vi "LogFile Schreiben.vi"(6 "Aktion":T1, 10 "LogFile erstellen?":bool) -> (0 "error out":errorcluster, 1 "Pfad+Name":path, 2 "Sequence":u32, 3 "LogFile schreiben ?":bool)   [LabVIEW 2020, in "LogKonfig.lvlib"]
uses:
  LogKonfig.lvlib
  Aktionen LogFile schreiben.ctl
  Aktionen Logdatei erstellen.ctl
  Log Sequence FGV Aktion.ctl
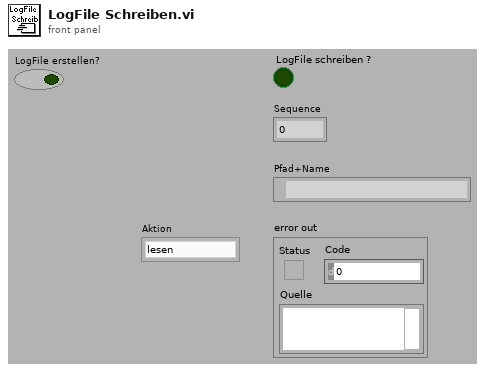
[diagram p1: front panel]
types:
  T1 = typedef "LogKonfig.lvlib/Aktionen LogFile schreiben.ctl" = enum16{"lesen", "schreiben", "initialisieren"}
  T2 = typedef "LogKonfig.lvlib/Log Sequence FGV Aktion.ctl" = enum16{"initialisieren", "lesen", "schreiben", "laden", "speichern", "übertragen"}
  T3 = typedef "LogKonfig.lvlib/Aktionen Logdatei erstellen.ctl" = enum16{"lesen", "Logdatei erstellen NEU", "Name NEU", "Pfad NEU", "Log Stop", "max Size"}
  T4 = typedef "TOOLweb Interface.lvlib/Typdefinitionen.lvlib/TOOLweb Signalverläufe.ctl" = waveform(dbl)[]
  T5 = cluster{"Index Array":i32[], "Namen Array":string[], "Spektrum File Name":bool}
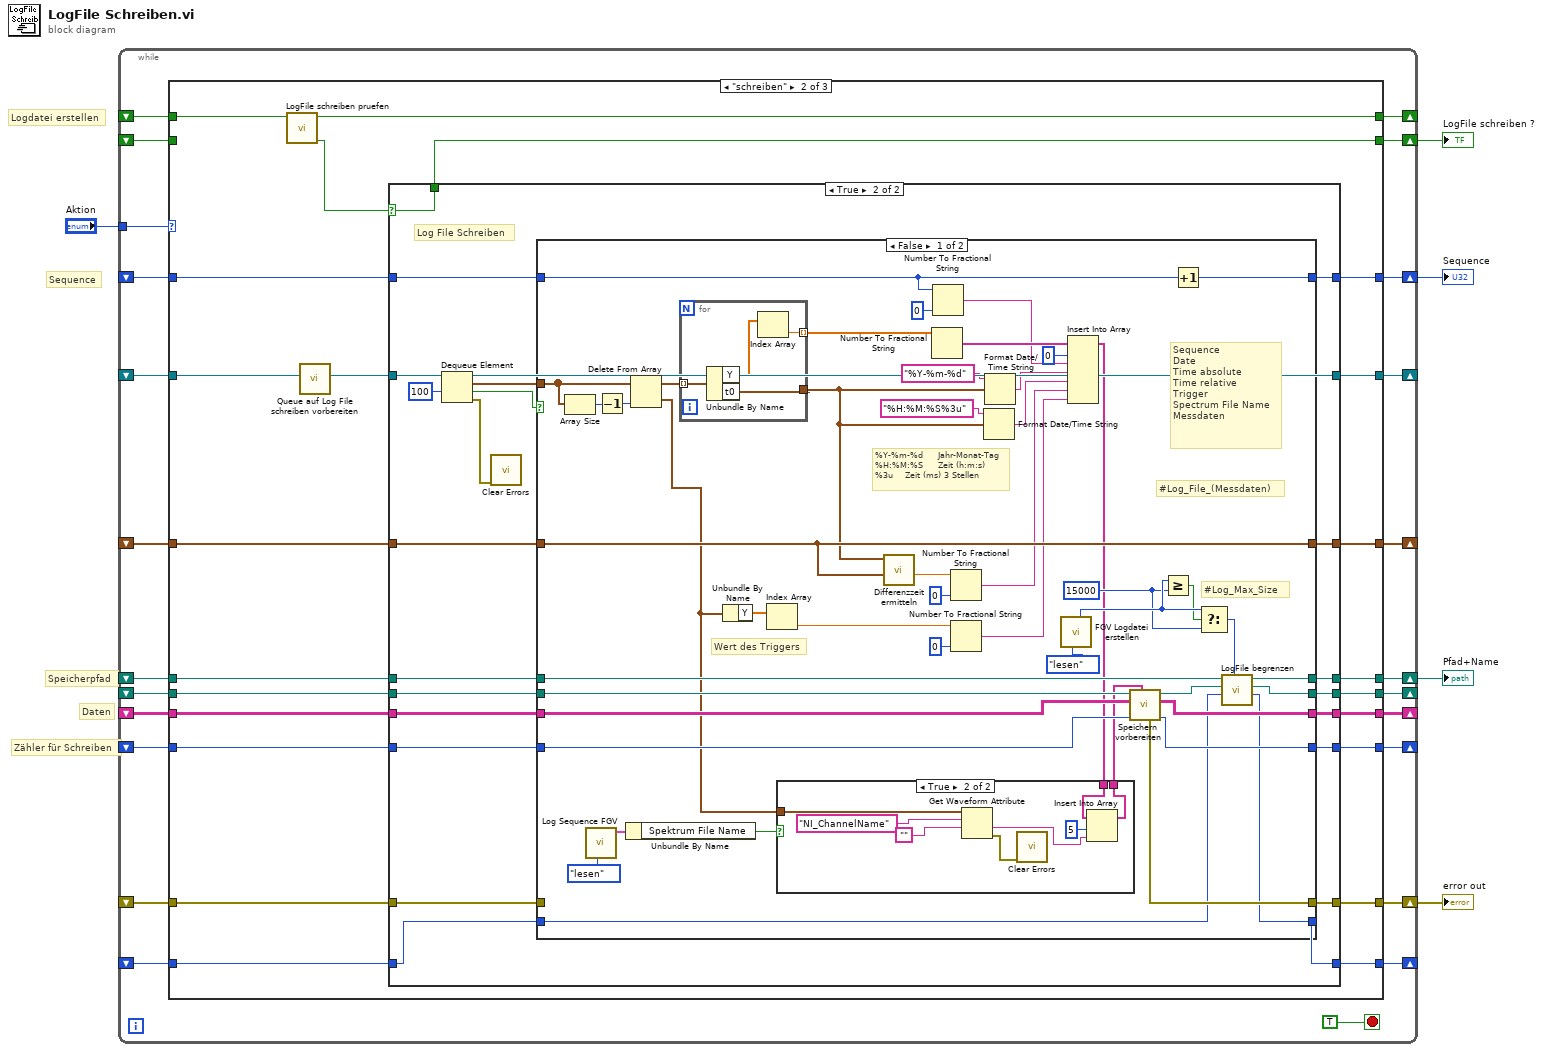
[diagram p0: block diagram]
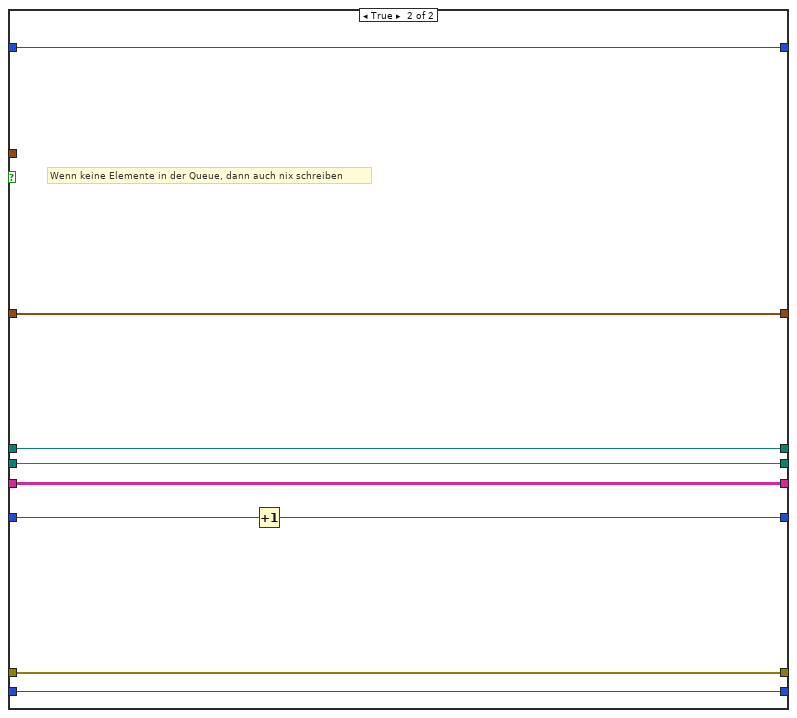
[diagram p5: hidden frame]
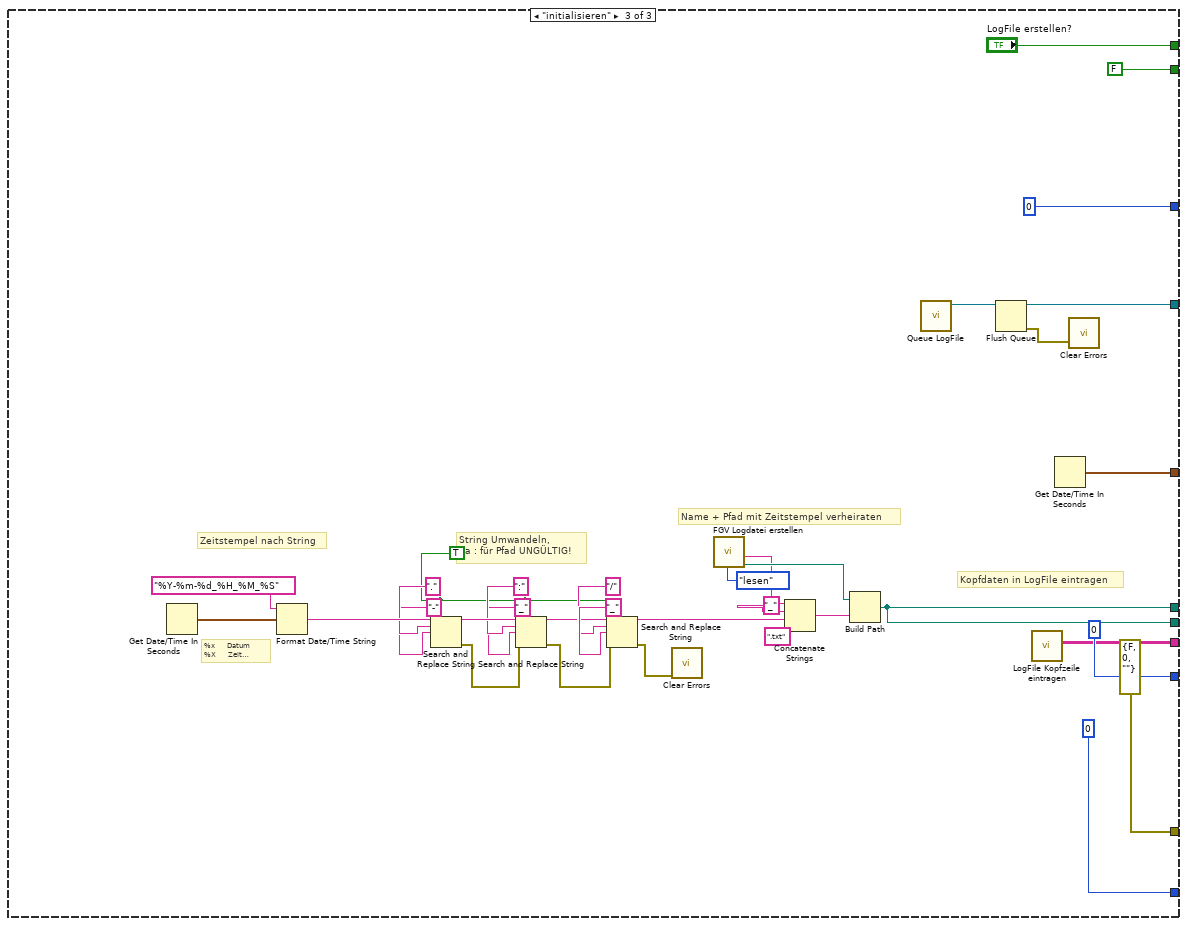
[diagram p6: hidden frame]
diagram:
  # "Zähler für Schreiben"
  # "Daten"
  # "Speicherpfad"
  # "Logdatei erstellen"
  # "Sequence"
  n1 = while {
    shift-right: [w28] -> _
    shift-left: _ -> [w29]
    shift-right: [w27] -> _
    shift-left: _ -> [w26]
    shift-right: [w25] -> _
    shift-left: _ -> [w24]
    shift-right: [w22] -> w3
    shift-left: _ -> [w23]
    tunnel: "Aktion" -> [w14]
    shift-right: [w20] -> _
    shift-left: _ -> [w19]
    shift-right: [w18] -> w4
    shift-left: _ -> [w17]
    shift-right: [w16] -> _
    shift-left: _ -> [w15]
    shift-right: [w13] -> w2
    shift-left: _ -> [w12]
    shift-right: [w11] -> w1
    shift-left: _ -> [w10]
    shift-right: [w9] -> _
    shift-left: _ -> [w8]
    shift-right: [w7] -> _
    shift-left: _ -> [w6]
    stop <- TRUE stop-if-true
    n2 = case shown="\"schreiben\"" w14 {
      tunnel: w29 -> [w36 w63 _]
      tunnel: [w36 w62 w184] -> w28
      tunnel: [w34 w61 i16 0 ("Index")] -> w27
      tunnel: w26 -> [w34 w60 _]
      tunnel: w17 -> [w37 w59 _]
      tunnel: [w38 w58 w182] -> w25
      tunnel: w24 -> [w38 w57 _]
      tunnel: w19 -> [w39 w49 _]
      tunnel: w23 -> [w40 w56 _]
      tunnel: [w40 w55 u32 0 ("Index")] -> w22
      tunnel: [w39 w53 w196] -> w20
      tunnel: [w37 w54 w166] -> w18
      tunnel: [w35 w46 "LogFile erstellen?"] -> w16
      tunnel: w15 -> [w35 w47 _]
      tunnel: [w33 w52 FALSE] -> w13
      tunnel: w12 -> [w33 _ _]
      tunnel: [w32 w51 errorcluster {"status"=FALSE, "code"=0, "source"=""} ("error out")] -> w11
      tunnel: w10 -> [w32 w50 _]
      tunnel: [w31 w43 i16 0 ("Index")] -> w9
      tunnel: w8 -> [w31 w44 _]
      tunnel: [w30 w42 w166] -> w7
      tunnel: w6 -> [w30 w41 _]
      frame "lesen", Default {
      }
      frame "schreiben" {
        n3 = call "LogFile schreiben pruefen.vi"("LogDatei erstellen"=w47) -> ("LogFile schreiben?"=w45:bool, "LogDatei erstellen"=w46:bool)  [unwired: 9 in]
        n4 = call "Queue auf Log File schreiben vorbereiten.vi"("Queue"=w49) -> ("Queue"=w48:refnum<queue>)  [unwired: 10 in]
        n5 = case shown="True" w45 {
          selector: w45 -> [w67 w82]
          tunnel: w63 -> [w69 w96]
          tunnel: [w69 w95] -> w62
          tunnel: [w68 w93] -> w61
          tunnel: w60 -> [w68 w92]
          tunnel: w59 -> [w70 w89]
          tunnel: [w71 w88] -> w58
          tunnel: w57 -> [w71 w87]
          tunnel: w48 -> [w72 w79]
          tunnel: w56 -> [w73 w86]
          tunnel: [w73 w85] -> w55
          tunnel: [w70 w84] -> w54
          tunnel: [w72 w83] -> w53
          tunnel: [w67 w82] -> w52
          tunnel: [w66 w81] -> w51
          tunnel: w50 -> [w66 w80]
          tunnel: w44 -> [w65 w77]
          tunnel: [w65 w76] -> w43
          tunnel: [w64 w75] -> w42
          tunnel: w41 -> [w64 w74]
          frame False {
            # "Wenn Log File nicht geschrieben werden soll, dann auch nix tun"
          }
          frame True {
            # "Log File Schreiben"
            n6 = Dequeue Element(queue=w79, timeout in ms (-1)=100 ("Timeout in ms(-1)")) -> (queue out=w83:refnum<queue>, element=w90:T4, timed out?=w91:bool, error out=w78:errorcluster)  [unwired: 1 in]
            n7 = call <vilib>:"Clear Errors.vi"("error in (no error)"=w78) -> ()  [unwired: 5 in, 2 out]
            n8 = case shown="False" w91 {
              tunnel: w96 -> [w124 w165]
              tunnel: [w122 w165] -> w95
              tunnel: w92 -> [w123 w161]
              tunnel: [w121 w160] -> w93
              tunnel: w90 -> [w133 _]
              tunnel: w89 -> [w114 w162]
              tunnel: [w128 w164] -> w88
              tunnel: w87 -> [w128 w164]
              tunnel: w86 -> [w137 w163]
              tunnel: [w139 w163] -> w85
              tunnel: [w119 w162] -> w84
              tunnel: [w120 w159] -> w81
              tunnel: w80 -> [_ w159]
              tunnel: w77 -> [w117 w158]
              tunnel: [w116 w158] -> w76
              tunnel: [w113 w157] -> w75
              tunnel: w74 -> [w118 w157]
              frame False {
                w108 = i64 15000 ("y")
                # "#Log_File_(Messdaten)"
                # "#Log_Max_Size"
                # "Wert des Triggers"
                # "Sequence\nDate\nTime absolute\nTime relative\nTrigger\nSpectrum File Name\nMessdaten"
                # "%Y-%m-%d     Jahr-Monat-Tag\n%H:%M:%S     Zeit (h:m:s)\n%3u    Zeit (ms) 3 Stellen"
                n9 = Array Size(array=w133) -> (size(s)=w134:i32)
                n10 = call "Log Sequence FGV.vi"("Aktion"=Log_Sequence_FGV_Aktion."lesen") -> ("Cluster (out)"=w98:T5)  [unwired: 10 in]
                n11 = Decrement(x=w134) -> (x-1=w131:i32)
                n12 = Unbundle By Name(w98) -> ("Spektrum File Name"=w97:bool)
                n13 = Delete From Array(array=w133, index=w131) -> (deleted portion=w100:waveform(dbl), array with subset deleted=w132:T4)  [unwired: 1 in]
                n14 = for {
                  tunnel: w132 -> [w153] mode=indexing
                  tunnel: [w156] -> w141 mode=indexing
                  tunnel: [w154] -> w103
                  n15 = Unbundle By Name(w153) -> ("Y"=w155:dbl[], "t0"=w154:timestamp)
                  n16 = Index Array(array=w155) -> (element=w156:dbl)  [unwired: 1 in]
                }
                n17 = Unbundle By Name(w100) -> ("Y"=w126:dbl[])
                n18 = Index Array(array=w126) -> (element=w125:dbl)  [unwired: 1 in]
                n19 = call "Differenzzeit ermitteln.vi"("Zeitstempel 2"=w128, "Zeitstempel 1"=w103) -> ("Differenzzeit in ms"=w130:sgl)  [unwired: 8 in, 1 out]
                n20 = Number To Fractional String(number=w141) -> (F-format string=w143:string[])  [unwired: 3 in]
                n21 = Number To Fractional String(number=w137, precision (6)=i16 0 ("Genauigkeit (6)")) -> (F-format string=w136:string)  [unwired: 2 in]
                n22 = Number To Fractional String(number=w130, precision (6)=i16 0 ("Genauigkeit (6)")) -> (F-format string=w106:string)  [unwired: 2 in]
                n23 = Number To Fractional String(number=w125, precision (6)=i16 0 ("Genauigkeit (6)")) -> (F-format string=w107:string)  [unwired: 2 in]
                n24 = Format Date/Time String(time format string (%c)="%H:%M:%S%3u" ("Zeitformatierungs-String (%c)"), seconds (now)=w103) -> (date/time string=w105:string)  [unwired: 1 in]
                n25 = Format Date/Time String(time format string (%c)="%Y-%m-%d" ("Zeitformatierungs-String (%c)"), seconds (now)=w103) -> (date/time string=w138:string)  [unwired: 1 in]
                n26 = call "FGV Logdatei erstellen.vi"("Aktion"=Aktionen_Logdatei_erstellen."lesen") -> ("max. Größe  in Byte neu"=w111:i64)  [unwired: 6 in, 4 out]
                n27 = Insert Into Array(array=w143, index=0 ("Index"), new element #1=w136, new element #2=w138, new element #3=w105, new element #4=w106, new element #5=w107) -> (w102:string[])
                n28 = case shown="True" w97 {
                  tunnel: w102 -> [w144 w151]
                  tunnel: [w144 w152] -> w101
                  tunnel: w100 -> [_ w146]
                  frame False {
                  }
                  frame True {
                    n29 = Get Waveform Attribute(5:"", 6:"NI_ChannelName", 7:w146) -> (0:w147:errorcluster, 1:w145:string)  [unwired: 1 in, 2 out]
                    n30 = call <vilib>:"Clear Errors.vi"("error in (no error)"=w147) -> ()  [unwired: 5 in, 2 out]
                    n31 = Insert Into Array(array=w151, index=5 ("Index"), new element=w145) -> (w152:string[])
                  }
                }
                n32 = call "Speichern vorbereiten.vi"("Neue Daten"=w101, "Index"=w123, "LogFile Daten"=w124, "Speicherpfad"=w118) -> ("Index"=w121:i16, "LogFile Daten"=w122:string[][], "Speicherpfad"=w115:path, "error out"=w120:errorcluster)  [unwired: 4 in]
                n33 = Greater Or Equal?(x=w111, y=w108) -> (x >= y?=w109:bool)
                n34 = Increment(x=w137) -> (x+1=w139:u32)
                n35 = Select(t=w111, s=w109, f=w108) -> (s? t:f=w110:i64)
                n36 = call "LogFile begrenzen.vi"("max. Größe  in Byte"=w110, "Index (Eingang)"=w117, "Pfad (Eingang)"=w115, "Pfad original (Eingang)"=w114) -> ("Index (Ausgang)"=w116:i16, "Pfad (Ausgang)"=w113:path, "Pfad original (Ausgang)"=w119:path)  [unwired: 5 in]
              }
              frame True {
                # "Wenn keine Elemente in der Queue, dann auch nix schreiben"
                n37 = Increment(x=w161) -> (x+1=w160:i16)
              }
            }
          }
        }
      }
      frame "initialisieren" {
        w176 = TRUE ("Alle ersetzen? (F)")
        # "Kopfdaten in LogFile eintragen"
        # "Name + Pfad mit Zeitstempel verheiraten"
        # "String Umwandeln, \nda : für Pfad UNGÜLTIG!"
        # "Zeitstempel nach String"
        # "%x      Datum\n%X      Zeit (h:m:s)"
        n38 = Get Date/Time In Seconds() -> (seconds since 1Jan1904=w193:timestamp)
        n39 = Format Date/Time String(time format string (%c)="%Y-%m-%d_%H_%M_%S" ("Zeitformatierungs-String (%c)"), seconds (now)=w193) -> (date/time string=w191:string)  [unwired: 1 in]
        n40 = Search and Replace String(replace all?=w176, input string=w191, search string="." ("Such-String"), replace string="-" ("String ersetzen(\"\")")) -> (result string=w188:string, error out=w171:errorcluster)  [unwired: 4 in, 2 out]
        n41 = Search and Replace String(replace all?=w176, input string=w188, search string=":" ("Such-String"), replace string="_" ("String ersetzen(\"\")"), error in=w171) -> (result string=w177:string, error out=w170:errorcluster)  [unwired: 3 in, 2 out]
        n42 = Search and Replace String(replace all?=w176, input string=w177, search string="/" ("Such-String"), replace string="_" ("String ersetzen(\"\")"), error in=w170) -> (result string=w175:string, error out=w169:errorcluster)  [unwired: 3 in, 2 out]
        n43 = call <vilib>:"Clear Errors.vi"("error in (no error)"=w169) -> ()  [unwired: 5 in, 2 out]
        n44 = call "FGV Logdatei erstellen.vi"("Aktion"=Aktionen_Logdatei_erstellen."lesen") -> ("Pfad LogDatei neu"=w185:path, "Name Log Datei neu"=w181:string)  [unwired: 6 in, 3 out]
        n45 = Concatenate Strings(w181, "_", w175, ".txt" ("String")) -> (w195:string)
        n46 = Build Path(base path=w185, name or relative path=w195) -> (appended path=w166:path)
        n47 = call "Queue LogFile.vi"() -> ("Queue (Ausgang)"=w197:refnum<queue>)  [unwired: 6 in, 1 out]
        n48 = Flush Queue(queue=w197) -> (queue out=w196:refnum<queue>, error out=w168:errorcluster)  [unwired: 1 in, 1 out]
        n49 = call "LogFile Kopfzeile eintragen.vi"() -> ("LogFile Kopfzeile"=w184:string[][])  [unwired: 11 in]
        n50 = Get Date/Time In Seconds() -> (seconds since 1Jan1904=w182:timestamp)
        n51 = call <vilib>:"Clear Errors.vi"("error in (no error)"=w168) -> ()  [unwired: 5 in, 2 out]
      }
    }
  }
  "Pfad+Name" <- w4
  "Sequence" <- w3
  "LogFile schreiben ?" <- w2
  "error out" <- w1
